vi "TEST - Wait on VIs Unloaded from Memory.vi"(8 "error in (no error)":errorcluster) -> (0 "error out":errorcluster, 2 "pass":bool)   [LabVIEW 2009]
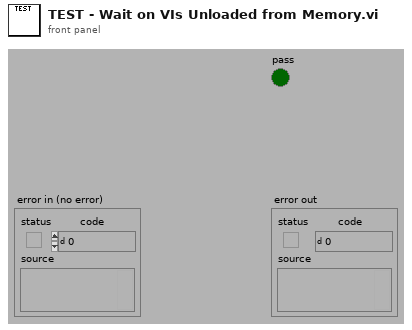
[diagram p1: front panel]
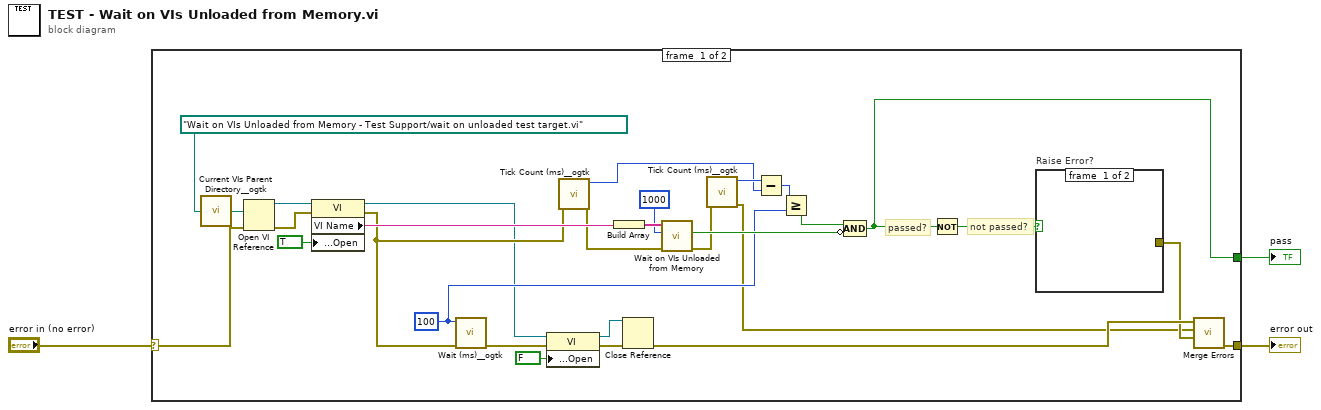
[diagram p0: block diagram]
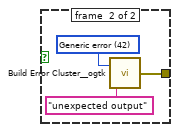
[diagram p2: hidden frame]
diagram:
  n1 = case shown="No Error" "error in (no error)" {
    selector: "error in (no error)" -> [w28 w36]
    tunnel: [w16 _] -> w3
    tunnel: [w32 w36] -> w1
    frame #0 {
      w14 = u32 100 ("milliseconds to wait")
      # "not passed?"
      # "passed?"
      n2 = call <userlib>:"Current VIs Parent Directory__ogtk.vi"("Relative path (.)"=path "Wait on VIs Unloaded from Memory - Test Support/wait on unloaded test target.vi") -> ("Parent Directory (+ Relative)"=w27:path)  [unwired: 4 in]
      n3 = Open VI Reference(vi path=w27, error in (no error)=w28) -> (vi reference=w22:refnum<vi>, error out=w12:errorcluster)  [unwired: 4 in]
      n4 = property class="VI"(reference=w22, error in=w12, "Front Panel.Open"=TRUE ("Front Panel Window:Open")) -> (reference out=w5:refnum<vi>, error out=w11:errorcluster, "VI Name"=w26:string)
      n5 = call <userlib>:"Wait (ms)__ogtk.vi"("error in (no error)"=w11, "milliseconds to wait"=w14) -> ("error out"=w7:errorcluster)  [unwired: 8 in, 1 out]
      n6 = property class="VI"(reference=w5, error in=w7, "Front Panel.Open"=FALSE ("Front Panel Window:Open")) -> (reference out=w4:refnum<vi>, error out=w6:errorcluster)
      n7 = call <userlib>:"Tick Count (ms)__ogtk.vi"("error in (no error)"=w11) -> ("error out"=w21:errorcluster, "millisecond timer value"=w17:u32)  [unwired: 9 in]
      n8 = Build Array(w26) -> (w25:string[])
      n9 = Close Reference(reference=w4, error in (no error)=w6) -> (error out=w30:errorcluster)
      n10 = call "Wait on VIs Unloaded from Memory.vi"("error in (no error)"=w21, "ms Timout (100ms)"=u32 1000, "VIs to Wait on"=w25) -> ("error out"=w20:errorcluster, "Timeout?"=w23:bool)  [unwired: 7 in]
      n11 = call <userlib>:"Tick Count (ms)__ogtk.vi"("error in (no error)"=w20) -> ("error out"=w8:errorcluster, "millisecond timer value"=w18:u32)  [unwired: 9 in]
      n12 = Subtract(x=w18, y=w17) -> (x-y=w15:u32)
      n13 = Greater Or Equal?(x=w15, y=w14) -> (x >= y?=w13:bool)
      n14 = Compound Arithmetic op=AND(w13, invert w23) -> (w16:bool)
      n15 = Not(x=w16) -> (.not. x?=w31:bool)
      n16 = case "Raise Error?" shown="True" w31 {
        tunnel: [_ w33] -> w19
        frame #0 {
        }
        frame #1 {
          w34 = 42 items=["No error", "Argument error", "Memory is full", "Out of zone", "End of file", "File already open", "Generic file I/O error", "File not found", "File permission error", "Disk is full", "Duplicate path", "Too many files open", "System feature not enabled", "Resource file not found", "Cannot add resource", "Resource not found", "Image not found", "Image memory error", "Pen does not exist", "Config type invalid", "Config token not found", "Config parse error", "Config memory error", "Bad external code format", "Bad external code offset", "External code not present", "Null window", "Destroy window error", "Null menu", "Print aborted", "Bad print record", "Print driver error", "Windows error during printing", "Memory error during printing", "Print dialog error", "Generic print error", "Invalid device refnum", "Device not found", "Device parameter error", "Device unit error", "Cannot open device", "Device call aborted", "Generic error", "Cancelled by user", "Object ID too low", "Object ID too high", "Object not in heap", "Unknown heap", "Unknown object (invalid DefProc)", "Unknown object (DefProc not in table)", "Message out of range", "Invalid (null) method", "Unknown message", "Manager call not supported", "Bad address", "Network operation in progress", "Network operation timed out", "Connection is busy", "Network attribute not supported", "Network error", "Address in use", "System out of memory", "Connection aborted", "Connection refused", "Not connected", "Already connected", "Connection closed", "Initialization error (interapplication manager)", "Bad occurrence", "Wait on unbound occurrence handler", "Occurrence queue overflow", "Datalog type conflict", "Unused", "Unrecognized type (interapplication manager)", "Memory corrupt", "Failed to make temporary DLL", "Old CIN version", "Drag socket not found", "Failed to load drop-object", "Failed to register OLE object", "Failed to release OLE object", "Format specifier type mismatch", "Unknown format specifier", "Too few format specifiers", "Too many format specifiers", "Scan failed", "Newer CIN version", "Error converting to variant", "Runtime menu error", "Password tampered", "Variant attribute not found", "Incompatible variant data type", "Event data is not available", "Event Store is not present", "Occurrence is not found", "Event Queue is not created", "Event info is not available", "Refnum passed is NULL", "Error retrieving Class GUID", "Error retrieving CoClass GUID", "Error retrieving TypeLib GUID.", "Bad built application magic bytes.", "Specific driver is different from the specific driver associated with the Logical Name.", "There is no session opened to the class driver.", "Max Error", "MAX - Error with config objects", "MAX - Error loading configuration", "MAX - Group not supported"]
          n17 = call <userlib>:"Build Error Cluster__ogtk.vi"("String to Prepend to source (\"\")"="unexpected output" ("String to Prepend to source (\"\")"), "code"=w34) -> ("error out"=w33:errorcluster)
        }
      }
      n18 = call <vilib>:"Merge Errors.vi"("error in 3 (no error)"=w19, "error in 2 (no error)"=w8, "error in 1 (no error)"=w30) -> ("error out"=w32:errorcluster)  [unwired: 4 in]
    }
    frame #1 {
    }
  }
  "pass" <- w3
  "error out" <- w1
